vi "$ICJC.vi"() -> (3 "字符串":string)   [LabVIEW 2016, in "环境动力监测库.lvlib" / "NMEA.lvlib"]
uses:
  NMEA.lvlib
panel:
  out "输出数组":u8[](array[numeric]) format="%02xH"
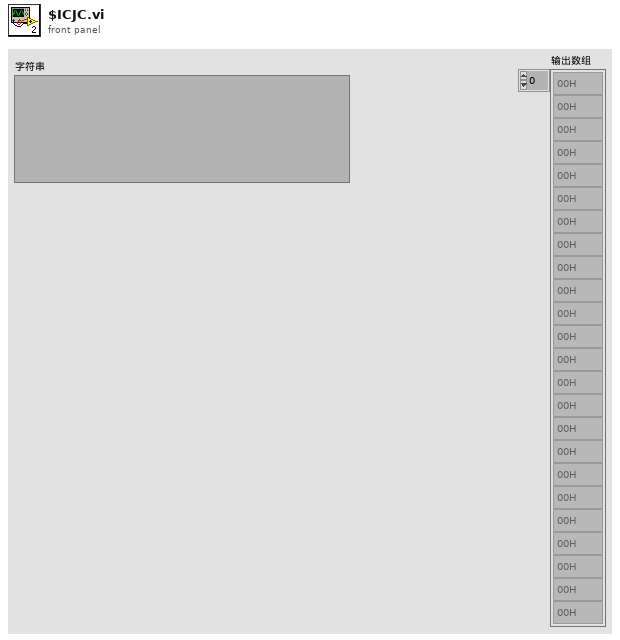
[diagram p1: front panel]
types:
  T1 = cluster{"指令/内容":string, "用户地址":string, "信息内容":u8[]}
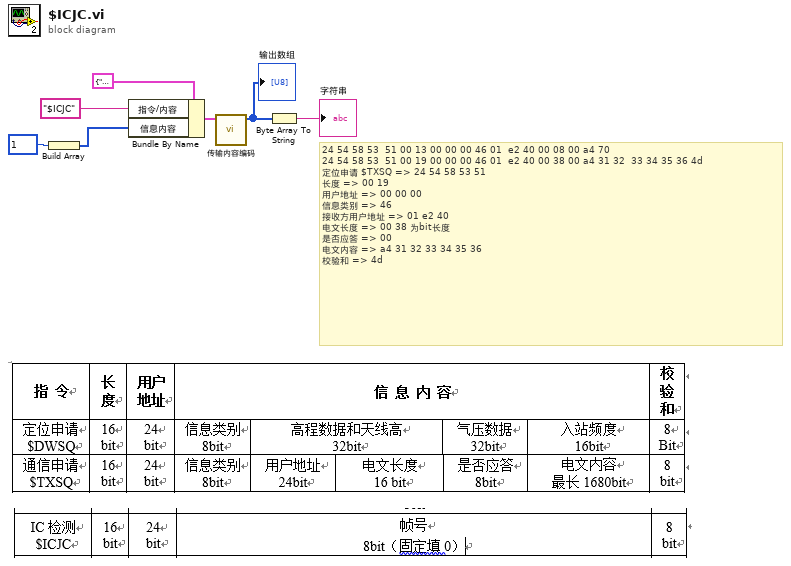
[diagram p0: block diagram]
diagram:
  # "24 54 58 53  51 00 13 00 00 00 46 01  e2 40 00 08 00 a4 70\n24 54 58 53  51 00 19 00 00 00 46 01  e2 40 00 38 00 a4 31 32  33 34 35 36 4d\n定位申请 $TXSQ => 24 54 58 53 51\n长度 => 00 19\n用户地址 => 00 00 00\n信息类别 => 46\n接收方用户地址 => 01 e2 40\n电文长度 => 00 38 为bit长度\n是否应答 => 00\n电文内容 => a4 31 32 33 34 35 36\n校验和 => 4d"
  n1 = Build Array(u8 1) -> (w4:u8[])
  n2 = Bundle By Name(cluster=T1 {"指令/内容"="", "用户地址"="", "信息内容"=[]} ("输入"), "指令/内容"="$ICJC" ("用户地址"), "信息内容"=w4) -> (w6:T1)
  n3 = call "传输内容编码.vi"("输入"=w6) -> ("输出数组"=w2:u8[])  [unwired: 10 in]
  "输出数组" <- w2
  n4 = Byte Array To String(unsigned byte array=w2) -> (string=→"字符串":string)
